vi "Agilent 66XX Series Take Measurement.vi"(0 "VISA resource name":refnum<visa-resource-name>, 1 "Current(0 Amps)":dbl format="%.3f", 2 "Location(Address 1)":u16(ring)=1 items=["Address 0", "Address 1", "Address 2", "Address 3", "Address 4 (not for 668x/669x/E4356a)"], 3 "Overvoltage prot value(50 Volts)":dbl=50.0 format="%.3f", 5 "Ouput(On:T)":bool=TRUE, 7 "Current Mode(Immediate:F)":bool, 9 "Voltage Mode(Immediate:F)":bool, 11 "error in (no error)":errorcluster, 12 "Voltage(0 Volts)":dbl format="%.3f", 13 "Trigger Delay(5000 ms)":u32=5000, 14 "Protection(None:0)":u16(ring) items=["None", "Overcurrent protection", "Overvoltage protection", "Overcurrent and overvoltage protection", "Clear overvoltage condition", "Clear overcurrent protection", "Set time delay"]) -> (15 "error out":errorcluster)   [LabVIEW 2012]
doc: "The Application Example configures, triggers (after a user defined time delay) and stores the setting to a user defined address."
uses:
  PowerSupply Control/Agilent 66XX Series.lvlib
panel:
  in  "Reset (F:no)":bool
  in  "ID query (T:yes)":bool=TRUE
  # "© 2005 National Instruments.  ALL RIGHTS RESERVED."
  # "Yes"
  # "No"
  # "Yes"
  # "No"
  # "Trigger"
  # "Immediate"
  # "Trigger"
  # "Immediate"
  # "On"
  # "Off"
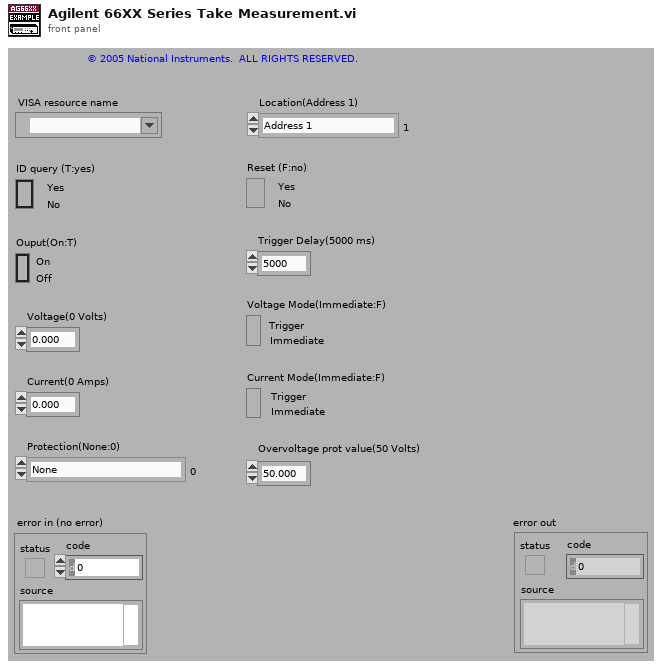
[diagram p1: front panel]
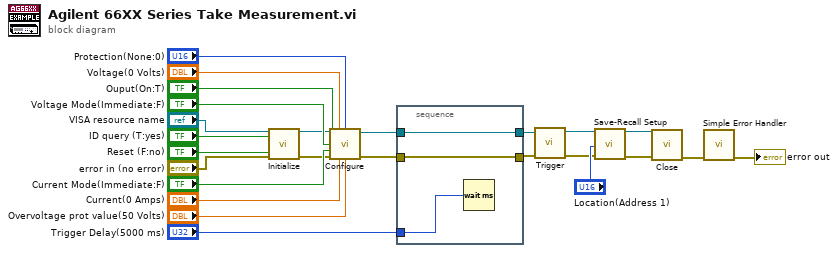
[diagram p0: block diagram]
diagram:
  n1 = call "Initialize.vi"("VISA resource name"="VISA resource name", "ID query (T:yes)"="ID query (T:yes)", "Reset (F:no)"="Reset (F:no)", "error in (no error)"="error in (no error)") -> ("VISA resource name out"=w10:refnum<visa-resource-name>, "error out"=w9:errorcluster)  [unwired: 10 in]
  n2 = call "Configure.vi"("VISA resource name"=w10, "Voltage(0 Volts)"="Voltage(0 Volts)", "Protection(None:0)"="Protection(None:0)", "Ouput(On:T)"="Ouput(On:T)", "Voltage Mode(F:Immediate)"="Voltage Mode(Immediate:F)", "Current Mode(F:Immediate)"="Current Mode(Immediate:F)", "error in (no error)"=w9, "Current(0 Amps)"="Current(0 Amps)", "Overvoltage prot value(50 Volts)"="Overvoltage prot value(50 Volts)") -> ("VISA resource name out"=w17:refnum<visa-resource-name>, "error out"=w16:errorcluster)  [unwired: 5 in]
  n3 = stacked-sequence {
    tunnel: w17 -> [w28]
    tunnel: w16 -> [w27]
    tunnel: [w28] -> w14
    tunnel: [w27] -> w15
    tunnel: "Trigger Delay(5000 ms)" -> [w26]
    frame #0 {
      n4 = Wait (ms)(milliseconds to wait=w26) -> ()  [unwired: 1 out]
    }
  }
  n5 = call "Trigger.vi"("VISA resource name"=w14, "error in (no error)"=w15) -> ("VISA resource name out"=w13:refnum<visa-resource-name>, "error out"=w12:errorcluster)  [unwired: 12 in]
  n6 = call "Save-Recall Setup.vi"("VISA resource name"=w13, "Address (0)"="Location(Address 1)", "error in (no error)"=w12) -> ("VISA resource name out"=w8:refnum<visa-resource-name>, "error out"=w7:errorcluster)  [unwired: 11 in]
  n7 = call "Close.vi"("VISA resource name"=w8, "error in (no error)"=w7) -> ("error out"=w2:errorcluster)  [unwired: 13 in]
  n8 = call <vilib>:"Simple Error Handler.vi"("error in (no error)"=w2) -> ("error out"=→"error out":errorcluster)  [unwired: 4 in, 4 out]
